vi "Gantry_Read-Write.vi"(0 "VISA resource name":refnum<visa-resource-name>="COM5", 7 "Command":string, 11 "error in (no error)":errorcluster, 12 "Open Serial":bool, 14 "Close Serial":bool) -> (2 "Warn(T)":bool, 3 "FH_NOT(T)":bool, 4 "VISA resource name out":refnum<visa-resource-name>="COM5", 6 "Response String Array":string[](array[string])=["01 0 OK IDLE WR 0"], 8 "Data":string, 10 "Warning Flags":string, 15 "error out":errorcluster={"status"=FALSE, "code"=1073481728, "source"="Zaber A Series.lvlib:Error Query.vi<ERR>\nInstrument 01 0 reports 1 warnings:  WR\r\n\r\n For warning explanations visit http://www.zaber.com/wiki/Manuals/ASCII_Protocol_Manual#Warning_Flags. \n\n\n<b>Complete call chain:</b>\r\n     Zaber A Series.lvlib:Error Query.vi\r\n     Zaber A Series.lvlib:Send Command.vi\r\n     Gantry_Read-Write.vi"})   [LabVIEW 2018]
doc: "This is a basic example demonstrating some of the low-level read and write VIs, with some example commands and a variety of output formats displayed."
uses:
  <vilib>/Utility/file.llb/Read Delimited Spreadsheet (string).vi
  Zaber A Series.lvlib
panel:
  out "Warn Desc":string
  out "Numeric":i32
  out "time(ms)":dbl=2.2750399999949878e-05
  out "Response Bundle Array":T1(array[cluster])=[{"Device"="01", "Axis"="0", "Reply Flag"="OK", "Status"="IDLE", "Warning Flags"="WR", "Data"="0"}]
  out "First Response Data Value":string="0"
  out "First Response Device Number":string="01"
  # "(c) 2017-2020 Zaber Technologies.  ALL RIGHTS RESERVED."
  # "https://www.zaber.com/protocol-manual?device=X-MCC4%20(rev%202)&peripheral=LSQ075D-E01T3A&version=7.21&protocol=ASCII#topic_scope"
  # "The purpose of this example is to show how you can enter commands and read back\nresponses. There are a number of ways to read responses, whether you just read one \nresponse, only want want part of the response, or prefer the complete string. Try writing\nsome of the example commands and see what response options are available. \n\nEnter the VISA resource your device is connected to and the Command string before running the VI."
  # "Example commands: \n'home' - device retracts to find the reference position\n'move rel 5000' - move the device by 5000 microsteps\n'01 get maxspeed' - returns the movement speed setting for device 1"
  # "If the command or data value you supply is not valid, you will get a warning message with a description of what the problem\nis in the error output."
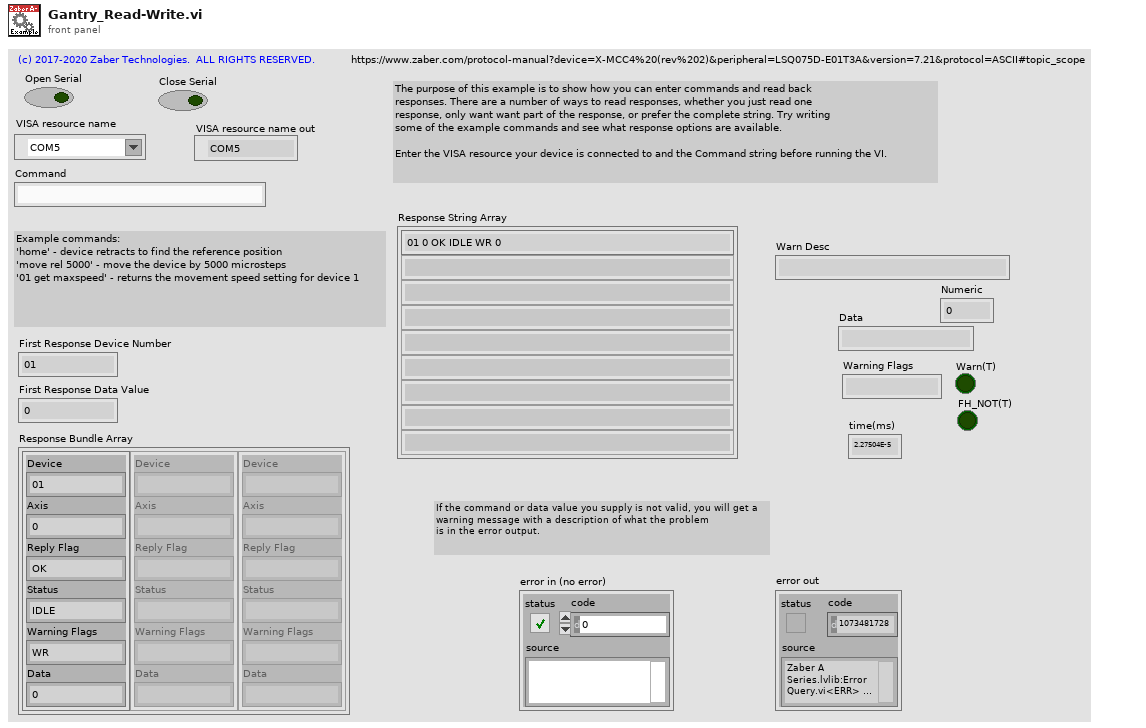
[diagram p1: front panel]
types:
  T1 = cluster{"Device":string, "Axis":string, "Reply Flag":string, "Status":string, "Warning Flags":string, "Data":string}[]
  T2 = cluster{"Device":string, "Axis":string, "Reply Flag":string, "Status":string, "Warning Flags":string, "Data":string}
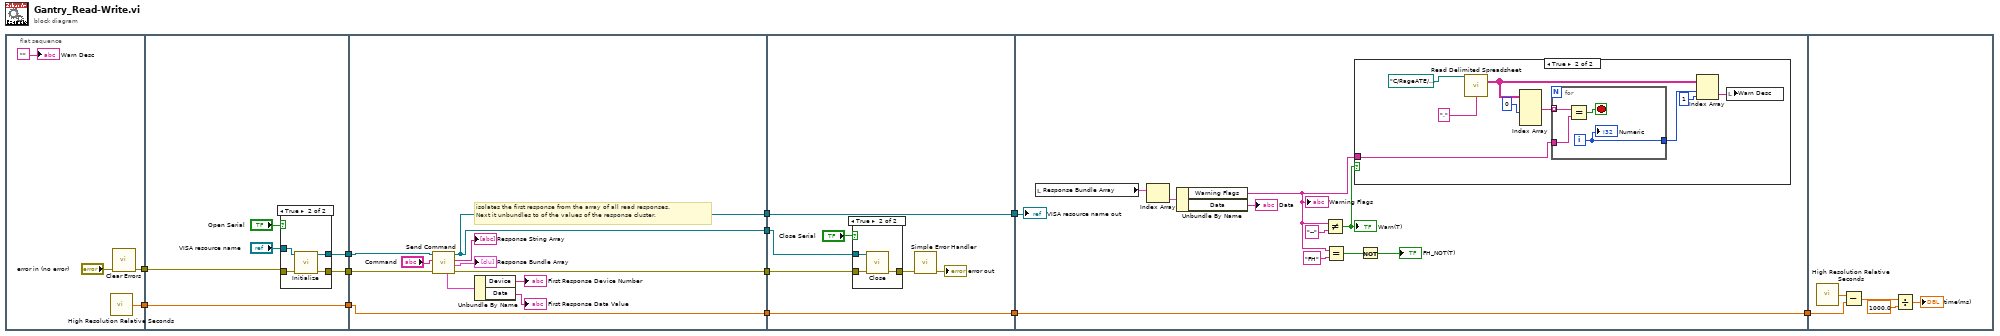
[diagram p0: block diagram]
diagram:
  n1 = flat-sequence {
    tunnel: [w16] -> w8
    tunnel: [w13] -> w1
    tunnel: [w19] -> w10
    tunnel: [w20] -> w9
    tunnel: w8 -> [w18]
    tunnel: [w18] -> w7
    tunnel: w1 -> [w17]
    tunnel: [w32] -> w12
    tunnel: [w29] -> w11
    tunnel: w10 -> [w34]
    tunnel: w9 -> [w33]
    tunnel: w7 -> [w30]
    tunnel: [w30] -> w6
    tunnel: [w29] -> w3
    tunnel: w12 -> [w45]
    tunnel: w11 -> [w44]
    tunnel: w6 -> [w41]
    tunnel: [w41] -> w5
    tunnel: [w40] -> w4
    tunnel: w3 -> [w40]
    tunnel: w5 -> [w60]
    tunnel: w4 -> [w61]
    tunnel: [w60] -> w2
    tunnel: w2 -> [w75]
    frame #0 {
      n2 = call <vilib>:"High Resolution Relative Seconds.vi"() -> ("relative seconds"=w16:dbl)
      n3 = call <vilib>:"Clear Errors.vi"("error in (no error)"="error in (no error)") -> ("error out"=w13:errorcluster)  [unwired: 5 in, 1 out]
      "Warn Desc" <- ""
    }
    frame #1 {
      n4 = case shown="True" "Open Serial" {
        tunnel: "VISA resource name" -> [w24 w28]
        tunnel: [w24 w27] -> w20
        tunnel: [w23 w26] -> w19
        tunnel: w17 -> [w23 w25]
        frame False {
        }
        frame True {
          n5 = call "Initialize.vi"("error in (no error)"=w25, "VISA resource name"=w28) -> ("error out"=w26:errorcluster, "VISA resource name out"=w27:refnum<visa-resource-name>)  [unwired: 8 in]
        }
      }
    }
    frame #2 {
      # "isolates the first response from the array of all read responses.\nNext it unbundles to of the values of the response cluster."
      n6 = call "Send Command.vi"("error in (no error)"=w34, "Command"="Command", "VISA resource name"=w33) -> ("error out"=w32:errorcluster, "Response Bundle Array"=→"Response Bundle Array":T1, "Response String Array"=→"Response String Array":string[], "VISA resource name out"=w29:refnum<visa-resource-name>, "First Response Bundle"=w39:T2)  [unwired: 3 in, 1 out]
      n7 = Unbundle By Name(w39) -> ("Device"=→"First Response Device Number":string, "Data"=→"First Response Data Value":string)
    }
    frame #3 {
      n8 = case shown="True" "Close Serial" {
        tunnel: [w47 w50] -> w46
        tunnel: w45 -> [w47 w49]
        tunnel: w44 -> [_ w48]
        frame False {
        }
        frame True {
          n9 = call "Close.vi"("error in (no error)"=w49, "VISA resource name"=w48) -> ("error out"=w50:errorcluster)  [unwired: 9 in]
        }
      }
      n10 = call <vilib>:"Simple Error Handler.vi"("error in (no error)"=w46) -> ("error out"=→"error out":errorcluster)  [unwired: 4 in, 4 out]
    }
    frame #4 {
      n11 = local read "Response Bundle Array"() -> (w59:T1)
      n12 = Index Array(array=w59) -> (element=w58:T2)  [unwired: 1 in]
      n13 = Unbundle By Name(w58) -> ("Warning Flags"=w52:string, "Data"=→"Data":string)
      "Warning Flags" <- w52
      n14 = Not Equal?(x=w52, y="--") -> (x != y?=w55:bool)
      "Warn(T)" <- w55
      n15 = Equal?(x=w52, y="FH") -> (x = y?=w54:bool)
      n16 = case shown="True" w55 {
        tunnel: w52 -> [_ w66]
        frame False {
        }
        frame True {
          n17 = call-poly <vilib>:"Read Delimited Spreadsheet.vi"("file path (dialog if empty)"=path "C:/RageATE/Instruments/Zaber Gantry/Zaber Labview Driver/RageATE-Zaber/Zaber-ErrorCodes.csv", "delimiter (\\t)"="," ("delimiter (\\t)")) -> ("all rows"=w65:string[][])  [unwired: 8 in, 5 out]
          n18 = Index Array(array=w65, index (col) #1=0 ("disabled index (col)")) -> (element #1=w67:string[])  [unwired: 3 in, 1 out]
          n19 = for {
            tunnel: w67 -> [w74] mode=indexing
            tunnel: w66 -> [w73]
            tunnel: [w71] -> w64
            i -> [w71]
            stop <- w72 stop-if-true
            n20 = Equal?(x=w74, y=w73) -> (x = y?=w72:bool)
            "Numeric" <- w71
          }
          n21 = Index Array(array=w65, index (row)=w64, index (col)=1 ("disabled index (col)")) -> (element=w62:string)
          n22 = local write "Warn Desc"(w62) -> ()
        }
      }
      n23 = Not(x=w54) -> (.not. x?=→"FH_NOT(T)":bool)
      "VISA resource name out" <- w61
    }
    frame #5 {
      n24 = call <vilib>:"High Resolution Relative Seconds.vi"() -> ("relative seconds"=w78:dbl)
      n25 = Subtract(x=w78, y=w75) -> (x-y=w77:dbl)
      n26 = Divide(x=w77, y=1000.0) -> (x/y=→"time(ms)":dbl)
    }
  }
